vi "testBlueTooth.vi"() -> ()   [LabVIEW 2011]
uses:
  <vilib>/NXT/NXT Controls/ConnectionType.ctl
panel:
  in  "Rudder":i32
  in  "Propeller":i32
  in  "Procedure":i32
  out "error out":errorcluster
  out "Is Paired with NXT?":bool
  in  "Connection type":T1
  in  "NXT name":string="Sasha Al"
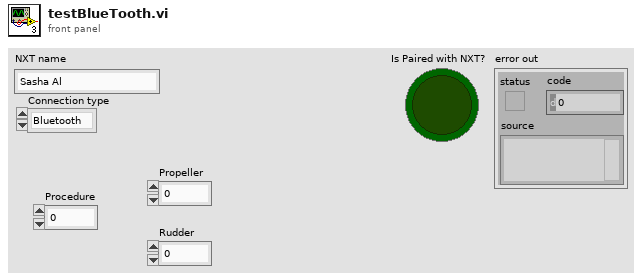
[diagram p1: front panel]
types:
  T1 = typedef "ConnectionType.ctl" = enum16{"Bluetooth", "USB", "WiFi"}
  T2 = typedef "nxt.ctl" = cluster{"nxtHandle":u32, "fileHandle":u32, "fileIterHandle":u32, "moduleHandle":u32, "modIterHandle":u32, "nxtIterHandle":u32}
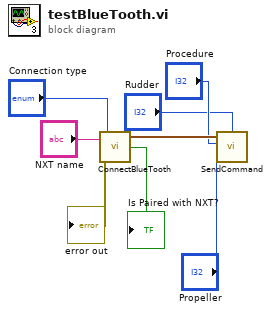
[diagram p0: block diagram]
diagram:
  n1 = call "ConnectBlueTooth.vi"("NXT name"="NXT name", "Connection type"="Connection type") -> ("NXTObject"=w8:T2, "Is Paired with NXT?"=→"Is Paired with NXT?":bool, "error out"=→"error out":errorcluster)
  n2 = call "SendCommand.vi"("Rudder"="Rudder", "Propeller"="Propeller", "Procedure"="Procedure", "NXTObject"=w8) -> ()
